vi "Displace-absolute.vi"(8 "error in (no error)":errorcluster, 9 "Min duration":dbl caption="Min. duration [s]", 10 "Position":dbl caption="Displacement [unit]", 11 "Motor-Maxon in":refnum<class "Motor-Maxon.lvclass">) -> (0 "error out":errorcluster, 3 "Motor-Maxon out":refnum<class "Motor-Maxon.lvclass">)   [LabVIEW 2013, in "PowderDeposition.lvlib" / "Motor-Maxon.lvclass"]
uses:
  Motor-Maxon.lvclass
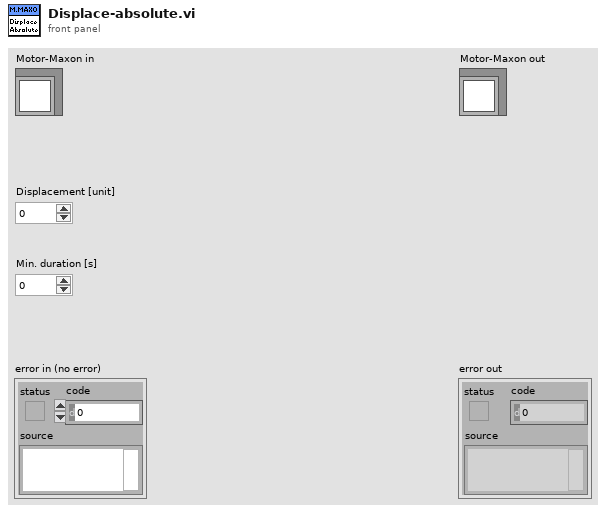
[diagram p1: front panel]
types:
  T1 = cluster{"profileVelocity":u32, "profileAcceleration":u32, "profileDeceleration":u32}
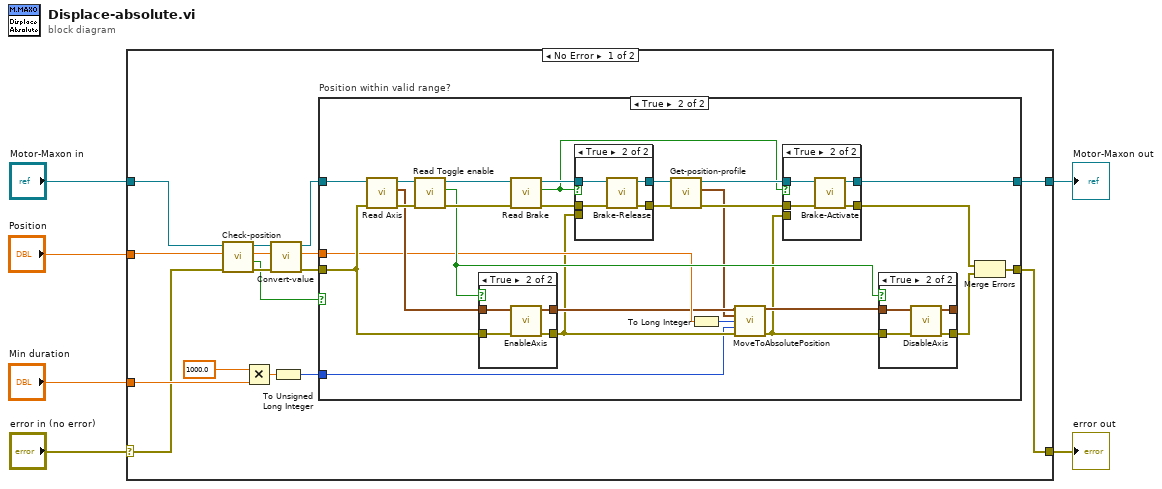
[diagram p0: block diagram]
diagram:
  n1 = case shown="No Error" "error in (no error)" {
    selector: "error in (no error)" -> [w7 w77]
    tunnel: [w14 w77] -> w5
    tunnel: [w22 w76] -> w3
    tunnel: "Motor-Maxon in" -> [w9 w76]
    tunnel: "Position" -> [w8 _]
    tunnel: "Min duration" -> [w11 _]
    frame No Error {
      n2 = call-dynamic "Check-position.vi"("error in (no error)"=w7, "Position in"=w8, "Motor-Serial in"=w9) -> ("error out"=w20:errorcluster, "In range?"=w16:bool, "Position out"=w21:dbl, "Motor-Serial out"=w17:refnum<class "Motor-Maxon.lvclass">)  [unwired: 5 in]
      n3 = Multiply(x=1000.0, y=w11) -> (x*y=w12:dbl)
      n4 = call-dynamic "Convert-value.vi"("error in (no error)"=w20, "Value in"=w21, "Motor-Serial in"=w17) -> ("error out"=w19:errorcluster, "Value out"=w15:dbl, "Motor-Serial out"=w18:refnum<class "Motor-Maxon.lvclass">)  [unwired: 6 in]
      n5 = To Unsigned Long Integer(number=w12) -> (unsigned 32bit integer=w10:u32)
      n6 = case "Position within valid range?" shown="True" w16 {
        tunnel: [w24 w35] -> w22
        tunnel: w19 -> [w23 w42]
        tunnel: w18 -> [w24 w41]
        tunnel: w15 -> [_ w36]
        tunnel: [w23 w34] -> w14
        tunnel: w10 -> [_ w25]
        frame False {
        }
        frame True {
          n7 = call-dynamic "Read Axis.vi"("error in (no error)"=w42, "Motor-Maxon in"=w41) -> ("error out"=w50:errorcluster, "Axis"=w49:cluster{"keyHandle":u32, "nodeID":u16}, "Motor-Maxon out"=w51:refnum<class "Motor-Maxon.lvclass">)  [unwired: 7 in]
          n8 = call-dynamic "Read Toggle enable.vi"("error in (no error)"=w50, "Motor-Maxon in"=w51) -> ("error out"=w47:errorcluster, "Toggle enable"=w37:bool, "Motor-Maxon out"=w48:refnum<class "Motor-Maxon.lvclass">)  [unwired: 7 in]
          n9 = case shown="True" w37 {
            tunnel: w49 -> [w71 w74]
            tunnel: w42 -> [w70 w75]
            tunnel: [w71 w73] -> w31
            tunnel: [w70 w72] -> w28
            frame False {
            }
            frame True {
              n10 = call <instrlib>:"EnableAxis.vi"("error in (no error)"=w75, "axis in"=w74) -> ("error out"=w72:errorcluster, "axis out"=w73:cluster{"keyHandle":u32, "nodeId":u16})  [unwired: 4 in]
            }
          }
          n11 = call-dynamic "Read Brake.vi"("error in (no error)"=w47, "Motor-Maxon in"=w48) -> ("error out"=w45:errorcluster, "Brake"=w38:bool, "Motor-Maxon out"=w46:refnum<class "Motor-Maxon.lvclass">)  [unwired: 7 in]
          n12 = case shown="True" w38 {
            tunnel: w46 -> [w65 w69]
            tunnel: w45 -> [w64 w68]
            tunnel: [w65 w67] -> w44
            tunnel: [w64 w66] -> w43
            tunnel: w28 -> [_ _]
            frame False {
            }
            frame True {
              n13 = call-dynamic "Brake-Release.vi"("error in (no error)"=w68, "Motor-Maxon in"=w69) -> ("error out"=w66:errorcluster, "Motor-Maxon out"=w67:refnum<class "Motor-Maxon.lvclass">)  [unwired: 8 in]
            }
          }
          n14 = call-dynamic "Get-position-profile.vi"("error in (no error)"=w43, "Motor-Maxon in"=w44) -> ("error out"=w39:errorcluster, "Position profile"=w26:T1, "Motor-Maxon out"=w40:refnum<class "Motor-Maxon.lvclass">)  [unwired: 7 in]
          n15 = To Long Integer(number=w36) -> (32bit integer=w27:i32)
          n16 = call <instrlib>:"MoveToAbsolutePosition.vi"("axis in"=w31, "position profile"=w26, "absolute position"=w27, "timeout"=w25, "error in (no error)"=w28) -> ("axis out"=w30:cluster{"keyHandle":u32, "nodeId":u16}, "error out"=w29:errorcluster)  [unwired: 9 in]
          n17 = case shown="True" w38 {
            tunnel: w40 -> [w53 w55]
            tunnel: w39 -> [w52 w54]
            tunnel: [w53 w56] -> w35
            tunnel: [w52 w57] -> w33
            tunnel: w29 -> [_ _]
            frame False {
            }
            frame True {
              n18 = call-dynamic "Brake-Activate.vi"("error in (no error)"=w54, "Motor-Maxon in"=w55) -> ("error out"=w57:errorcluster, "Motor-Maxon out"=w56:refnum<class "Motor-Maxon.lvclass">)  [unwired: 8 in]
            }
          }
          n19 = case shown="True" w37 {
            tunnel: w30 -> [w59 w60]
            tunnel: w29 -> [w58 w61]
            tunnel: [w59 w63] -> _
            tunnel: [w58 w62] -> w32
            frame False {
            }
            frame True {
              n20 = call <instrlib>:"DisableAxis.vi"("error in (no error)"=w61, "axis in"=w60) -> ("error out"=w62:errorcluster, "axis out"=w63:cluster{"keyHandle":u32, "nodeId":u16})  [unwired: 4 in]
            }
          }
          n21 = Merge Errors(w33, w32) -> (w34:errorcluster)
        }
      }
    }
    frame Error {
    }
  }
  "error out" <- w5
  "Motor-Maxon out" <- w3
